vi "RPC Remote Call.vi"(5 "IP (\"\")":string) -> (2 "Remote Call?":bool)   [LabVIEW 2011]
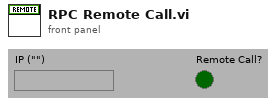
[diagram p1: front panel]
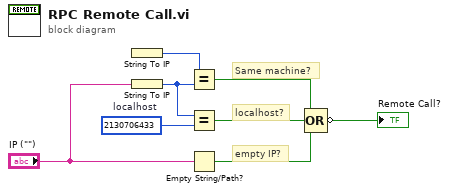
[diagram p0: block diagram]
diagram:
  w4 = u32 2130706433  # localhost
  # "empty IP?"
  # "localhost?"
  # "Same machine?"
  n1 = String To IP() -> (0:w6:u32)  [unwired: 1 out]
  n2 = String To IP(1:"IP (\"\")") -> (0:w5:u32)
  n3 = Equal?(x=w6, y=w5) -> (x = y?=w8:bool)
  n4 = Equal?(x=w5, y=w4) -> (x = y?=w3:bool)
  n5 = Empty String/Path?(string/path="IP (\"\")") -> (empty?=w2:bool)
  n6 = Compound Arithmetic op=OR(w8, w3, w2) -> (invert →"Remote Call?":bool)
